vi "Create User Event - Stop.vi"(8 "error in (no error)":T1 caption="Fehler (Eingang, kein Fehler)") -> (0 "error out":T1 caption="Fehler (Ausgang)", 2 "Benutzerereignis - Stopp":refnum<user-event>, 3 "Stoppereignisregistrierung (Referenz)":refnum<event-registration>)   [LabVIEW 2014, in "MyQH User Event - Stop.lvlib"]
doc: "Erstellt ein boolesches Benutzerereignis, mit dem die Ereignisschleife der Schleife zur Nachrichtenbehandlung gestoppt wird."
uses:
  MyQH User Event - Stop.lvlib
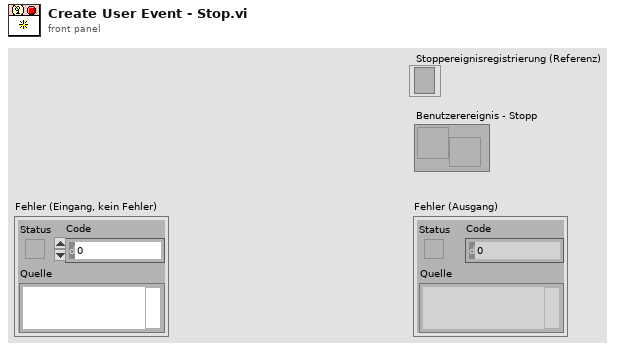
[diagram p1: front panel]
types:
  T1 = cluster{"Status":bool, "Code":i32, "Quelle":string}
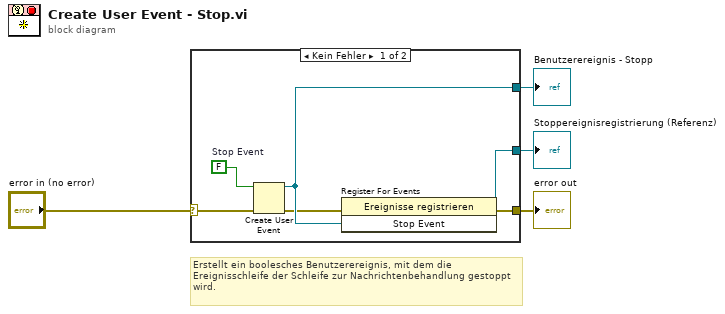
[diagram p0: block diagram]
diagram:
  # "Erstellt ein boolesches Benutzerereignis, mit dem die Ereignisschleife der Schleife zur Nachrichtenbehandlung gestoppt wird."
  n1 = case shown="Kein Fehler" "error in (no error)" {
    selector: "error in (no error)" -> [w5 w11]
    tunnel: [w10 _] -> w4
    tunnel: [w9 _] -> w3
    tunnel: [w6 w11] -> w2
    frame No Error {
      w8 = FALSE  # Stop Event
      n2 = Create User Event(user event datatype=w8, error in=w5) -> (user event=w10:refnum<user-event>, error out=w7:errorcluster)
      n3 = register-events(error in=w7, w10) -> (reference out=w9:refnum<event-registration>, error out=w6:errorcluster)  [unwired: 1 in]
    }
    frame Error {
    }
  }
  "Benutzerereignis - Stopp" <- w4
  "error out" <- w2
  "Stoppereignisregistrierung (Referenz)" <- w3
